vi "convert.vi"(1 "String":string) -> (0 "Numeric":dbl)   [LabVIEW 2018]
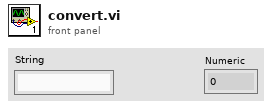
[diagram p1: front panel]
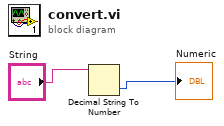
[diagram p0: block diagram]
diagram:
  n1 = Decimal String To Number(string="String") -> (number=→"Numeric":i32)  [unwired: 2 in, 1 out]
